vi "Test DAQmx Bus Analog Input and Output.vi"() -> ()   [LabVIEW 2021]
uses:
  <vilib>/TSA/Omni-Bus/Omni-Bus/Omni_Bus.lvclass
  <vilib>/TSA/Omni-Bus/Omni-Bus/Support/Broad Types.ctl
  <vilib>/TSA/Abstract Data Classes/Abs_Types/Type/Abs_Type.lvclass/Abs_Type.ctl
  <vilib>/TSA/Omni-Bus/Omni-Bus/Omni_Bus.lvclass/Omni_Bus.ctl
  <vilib>/TSA/Omni-Bus/Omni-Bus/Support/Write/Write DBL.vi
  <vilib>/TSA/Omni-Bus/Omni-Bus/Support/Read/Read DBL.vi
  <vilib>/TSA/Omni-Bus/Omni-Bus/Support/FindVar.vi
  <vilib>/Utility/error.llb/Clear Errors.vi
  <vilib>/TSA/Omni-Bus/Omni-Bus/Properties/Read Var Map.vi
  <vilib>/TSA/Abstract Data Classes/Abs_Types/Type/Properties/Read Tag.vi
  Source/DAQmx-Bus.lvclass
  C:/Program Files (x86)/National Instruments/LabVIEW 2021/vi.lib/TSA/Omni-Bus/Omni-Bus/Bus Access/Bus_Access.lvclass
  <vilib>/TSA/Abstract Data Classes/Abs_Types/Double Float/Abs_Double Float.lvclass
  C:/Program Files (x86)/National Instruments/LabVIEW 2021/vi.lib/TSA/Abstract Data Classes/Abs_Types/Type/Abs_Type.lvclass
  <vilib>/TSA/Abstract Data Classes/Abs_Types/Value/Abs_Value.lvclass
  <vilib>/TSA/Omni-Bus/Omni-Bus/Support/Check For Read Only Error.vi
  <vilib>/TSA/Omni-Bus/Omni-Bus/Support/Incorrect Tag String Error.vi
  <vilib>/TSA/Abstract Data Classes/Abs_Types/Type/Abs_Type.lvclass
panel:
  out "Gauge":dbl(knob) scale=-5.0..5.0
  in  "Combo Box 2":string(combo)
  in  "Slide":dbl(slide) scale=-5.0..5.0
  out "timed out?":bool
  in  "stop":bool
  in  "Combo Box":string(combo)
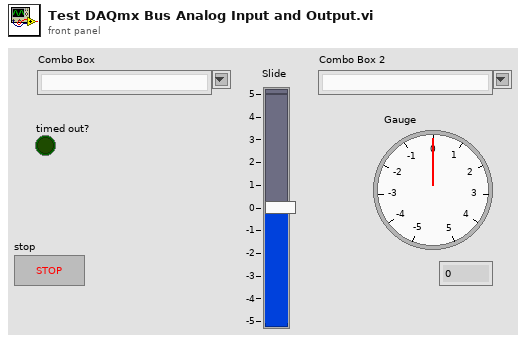
[diagram p1: front panel]
types:
  T1 = typedef "Omni_Bus.lvclass/Broad Types.ctl" = enum16{"All Tags", "NI Specific Type", "Boolean", "String", "Numeric", "Float", "Integer", "Collection", "All Value Types", "Non Value Types"}
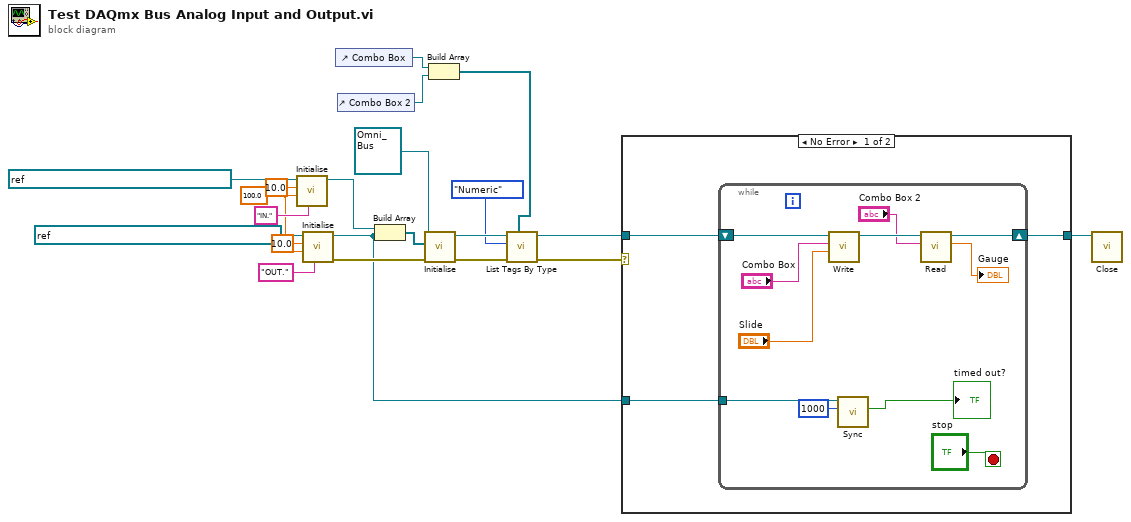
[diagram p0: block diagram]
diagram:
  w1 = 100.0 ("Update Rate (Hz) - Non HW Timed")
  n1 = call "Initialise.vi"("Tag Root"="IN.", "Update Rate (Hz) - Non HW Timed"=w1, "timeout (s)"=10.0 ("timeout"), "DAQmx Task"=refnum<k21> "Single Sample Analog In On Demand" ("DAQmx Device")) -> ("DAQmx-Bus out"=w8:refnum<class "DAQmx-Bus.lvclass">)  [unwired: 6 in, 1 out]
  n2 = call "Initialise.vi"("Tag Root"="OUT.", "Update Rate (Hz) - Non HW Timed"=w1, "timeout (s)"=10.0 ("timeout"), "DAQmx Task"=refnum<k21> "Single Sample Analog Output Ondemand" ("DAQmx Device")) -> ("error out"=w18:errorcluster, "DAQmx-Bus out"=w11:refnum<class "DAQmx-Bus.lvclass">)  [unwired: 6 in]
  n3 = control-ref of="Combo Box"() -> (w4:refnum<vi>)
  n4 = control-ref of="Combo Box 2"() -> (w3:refnum<vi>)
  n5 = Build Array(w8, w11) -> (w20:refnum<class "DAQmx-Bus.lvclass">[])
  n6 = call-dynamic "Initialise.vi"("error in (no error)"=w18, "Bus Access"=w20, "Var Bus in"=refnum<class "Omni_Bus.lvclass"> refnum) -> ("error out"=w15:errorcluster, "Var Bus out"=w16:refnum<class "Omni_Bus.lvclass">)  [unwired: 7 in]
  n7 = Build Array(w4, w3) -> (w2:refnum<vi>[])
  n8 = call <vilib>:"List Tags By Type.vi"("Combo Boxes"=w2, "error in (no error)"=w15, "Broad Types"=Broad_Types."Numeric", "Var Bus in"=w16) -> ("error out"=w13:errorcluster, "Var Bus out"=w14:refnum<class "Omni_Bus.lvclass">)  [unwired: 4 in, 2 out]
  n9 = case shown="No Error" w13 {
    tunnel: [w24 w36] -> w17
    tunnel: w14 -> [w23 w36]
    tunnel: w11 -> [w22 _]
    frame No Error {
      n10 = while {
        shift-right: [w27] -> w24
        shift-left: w23 -> [w35]
        tunnel: w22 -> [w32]
        stop <- "stop" stop-if-true
        n11 = call-poly <vilib>:"Write.vi"("Numeric"="Slide", "Tag"="Combo Box", "Omni_Bus in"=w35) -> ("Omni_Bus out"=w28:refnum<class "Omni_Bus.lvclass">)  [unwired: 7 in, 1 out]
        n12 = call-dynamic "Sync.vi"("timeout in ms (-1)"=1000, "DAQmx-Bus in"=w32) -> ("timed out?"=→"timed out?":bool)  [unwired: 7 in, 2 out]
        n13 = call-poly <vilib>:"Read.vi"("Tag"="Combo Box 2", "Var Bus in"=w28) -> ("Numeric"=→"Gauge":dbl, "Var Bus out"=w27:refnum<class "Omni_Bus.lvclass">)  [unwired: 7 in, 1 out]
      }
    }
    frame Error {
    }
  }
  n14 = call-dynamic "Close.vi"("Data in"=w17) -> ()  [unwired: 9 in, 2 out]
